vi "Open_Top_Level_VIs.vi"(8 "error in (no error)":errorcluster, 11 "Build in":refnum<class "AB_Targetfile.lvclass">) -> (0 "error out":errorcluster, 2 "Top-Level VIs":refnum<vi>[](array[refnum]), 3 "Build out":refnum<class "AB_Targetfile.lvclass">)   [LabVIEW 2020, in "AB_Targetfile.lvclass"]
uses:
  <vilib>/AppBuilder/AB_Classes/TargetFile/AB_Targetfile.lvclass
  <vilib>/AppBuilder/AB_Classes/Build/AB_Build.lvclass
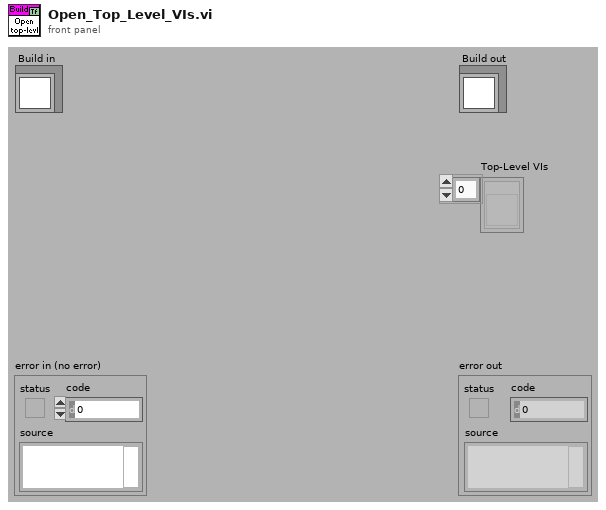
[diagram p1: front panel]
types:
  T1 = enum32{"Bad", "Idle", "Run top level", "Running"}
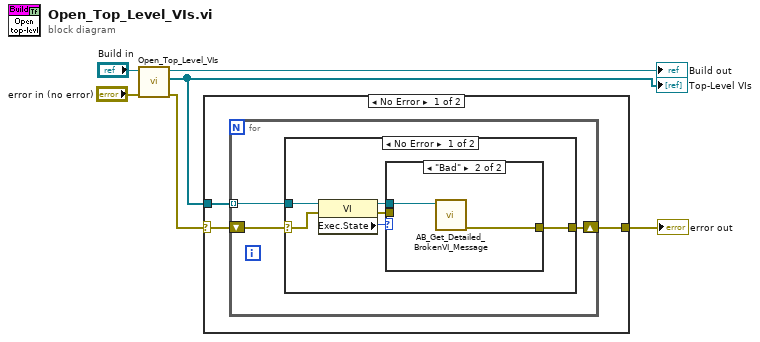
[diagram p0: block diagram]
diagram:
  n1 = call-parent "Open_Top_Level_VIs.vi"("error in (no error)"="error in (no error)", "Build in"="Build in") -> ("error out"=w2:errorcluster, "Top-Level VIs"=w3:refnum<vi>[], "Build out"=→"Build out":refnum<class "AB_Targetfile.lvclass">)  [unwired: 7 out]
  "Top-Level VIs" <- w3
  n2 = case shown="No Error" w2 {
    selector: w2 -> [w9 w23]
    tunnel: [w8 w23] -> w1
    tunnel: w3 -> [w7 _]
    frame No Error {
      n3 = for {
        shift-right: [w12] -> w8
        shift-left: w9 -> [w11]
        tunnel: w7 -> [w10] mode=indexing
        n4 = case shown="No Error" w11 {
          selector: w11 -> [w18 w22]
          tunnel: [w15 w22] -> w12
          tunnel: w10 -> [w13 _]
          frame No Error {
            n5 = property class="VI"(reference=w13, error in=w18) -> (reference out=w16:refnum<vi>, error out=w14:errorcluster, "Exec.State"=w17:T1)
            n6 = case shown="\"Bad\"" w17 {
              tunnel: w16 -> [_ w21]
              tunnel: [w19 w20] -> w15
              tunnel: w14 -> [w19 _]
              frame Default {
              }
              frame "Bad" {
                n7 = call <vilib>:"AB_Get_Detailed_BrokenVI_Message.vi"("VI refnum"=w21) -> ("error out"=w20:errorcluster)  [unwired: 10 in]
              }
            }
          }
          frame Error {
          }
        }
      }
    }
    frame Error {
    }
  }
  "error out" <- w1
